vi "GetNumber.vi"(8 "error in (no error)":errorcluster, 11 "ExampleClass in":refnum<class "ExampleClass.lvclass">) -> (0 "error out":errorcluster, 2 "Number":i32, 3 "ExampleClass out":refnum<class "ExampleClass.lvclass">)   [LabVIEW 2012, in "ExampleClass.lvclass"]
uses:
  ExampleClass.lvclass
  ExampleClass.lvclass/ExampleClass.ctl
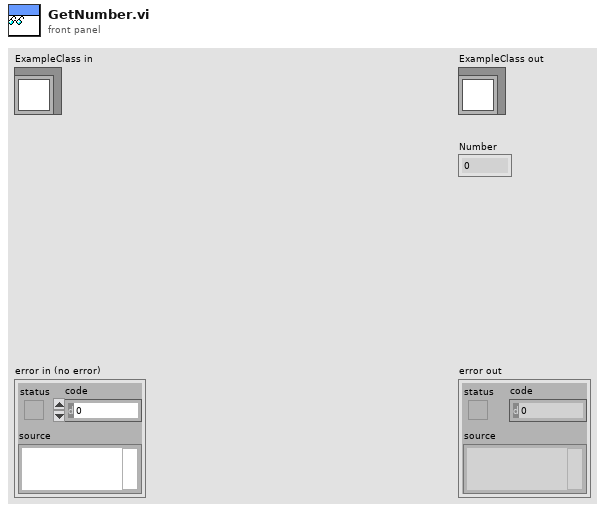
[diagram p1: front panel]
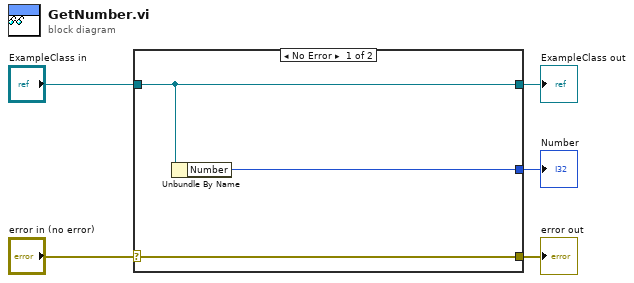
[diagram p0: block diagram]
diagram:
  n1 = case shown="No Error" "error in (no error)" {
    selector: "error in (no error)" -> [w8 w9]
    tunnel: [w8 w9] -> w4
    tunnel: [w7 w10] -> w2
    tunnel: "ExampleClass in" -> [w7 w10]
    tunnel: [w6 _] -> w1
    frame No Error {
      n2 = Unbundle By Name(w7) -> ("Number"=w6:i32)
    }
    frame Error {
    }
  }
  "error out" <- w4
  "ExampleClass out" <- w2
  "Number" <- w1
